vi "Clock.vi"() -> (2 "SYS Current Time":dbl format="%.3f")   [LabVIEW 2018]
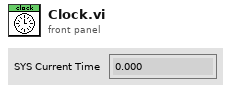
[diagram p1: front panel]
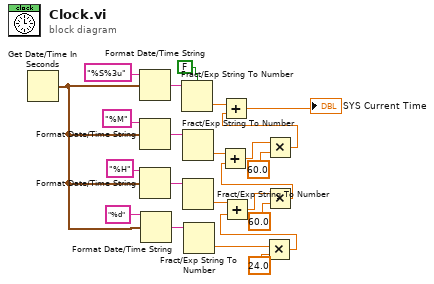
[diagram p0: block diagram]
diagram:
  n1 = Get Date/Time In Seconds() -> (seconds since 1Jan1904=w9:timestamp)
  n2 = Format Date/Time String(time format string (%c)="%S%3u", seconds (now)=w9) -> (date/time string=w23:string)  [unwired: 1 in]
  n3 = Format Date/Time String(time format string (%c)="%M", seconds (now)=w9) -> (date/time string=w18:string)  [unwired: 1 in]
  n4 = Format Date/Time String(time format string (%c)="%H", seconds (now)=w9) -> (date/time string=w17:string)  [unwired: 1 in]
  n5 = Format Date/Time String(time format string (%c)="%d", seconds (now)=w9) -> (date/time string=w10:string)  [unwired: 1 in]
  n6 = Fract/Exp String To Number(use system decimal point (T)=FALSE, string=w23) -> (number=w3:dbl)  [unwired: 2 in, 1 out]
  n7 = Fract/Exp String To Number(string=w18) -> (number=w16:dbl)  [unwired: 3 in, 1 out]
  n8 = Fract/Exp String To Number(string=w17) -> (number=w8:dbl)  [unwired: 3 in, 1 out]
  n9 = Fract/Exp String To Number(string=w10) -> (number=w6:dbl)  [unwired: 3 in, 1 out]
  n10 = Multiply(x=w6, y=24.0) -> (x*y=w4:dbl)
  n11 = Add(x=w8, y=w4) -> (x+y=w7:dbl)
  n12 = Multiply(x=w7, y=60.0) -> (x*y=w15:dbl)
  n13 = Add(x=w16, y=w15) -> (x+y=w14:dbl)
  n14 = Multiply(x=w14, y=60.0) -> (x*y=w2:dbl)
  n15 = Add(x=w3, y=w2) -> (x+y=→"SYS Current Time":dbl)
